vi "Destroy Request Events.vi"(8 "error in (no error)":errorcluster) -> (0 "error out":errorcluster)   [LabVIEW 2015, in "Tool Module.lvlib"]
doc: "Destroy the requests user events, even if there is an incoming error.\n\n<b>NOTE</b>: The contents of this VI are automatically generated and modified by the <b>Tools > Delacor > DQMH</b> utilities. Consider using those utilities instead of making your own modifications to this VI.\n_____\nBased on Delacor QMH Project Template 2.1.0.2."
uses:
  Tool Module.lvlib
panel:
  # "NOTE: The contents of this VI are automatically generated and modified by the Tools > Delacor > DQMH utilities. Consider using those utilities instead of making your own modifications to this VI."
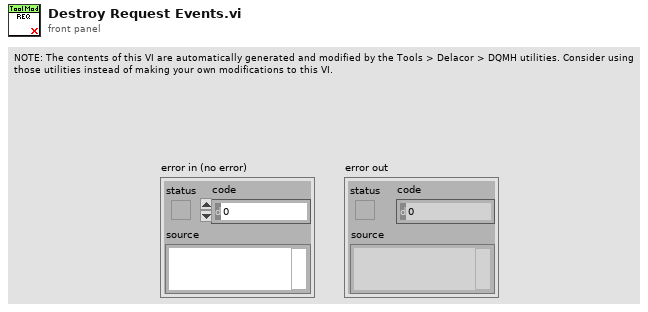
[diagram p1: front panel]
types:
  T1 = typedef "Tool Module.lvlib/Request Events--cluster.ctl" = cluster{"Stop Module":refnum<user-event>, "Show Panel":refnum<user-event>, "Hide Panel":refnum<user-event>, "Get Module Execution Status":refnum<user-event>, "Show Diagram":refnum<user-event>, "Test Trig 2":refnum<user-event>, "GOTO":refnum<user-event>, "Start Inspect":refnum<user-event>, "CONNECT":refnum<user-event>, "Get All Inspect Data":refnum<user-event>, "Get Inspection Limits":refnum<user-event>, "Set Inspection Limits":refnum<user-event>, "Update Status":refnum<user-event>, "Start Data Monitor":refnum<user-event>, "Get FPGA Setup Params":refnum<user-event>, "Set FPGA Setup Params":refnum<user-event>, "Set Tool Config":refnum<user-event>, "Get Tool Config":refnum<user-event>, "Set Integration Count":refnum<user-event>, "Set Laser Params":refnum<user-event>, "Get Mtrl Ctrl Reg":refnum<user-event>, "Commit Ctrl Reg":refnum<user-event>, "Set Event Logger":refnum<user-event>, "Write to File":refnum<user-event>, "Read from File":refnum<user-event>, "Set Device Temp Thresholds":refnum<user-event>, "Get Cycle Count":refnum<user-event>}
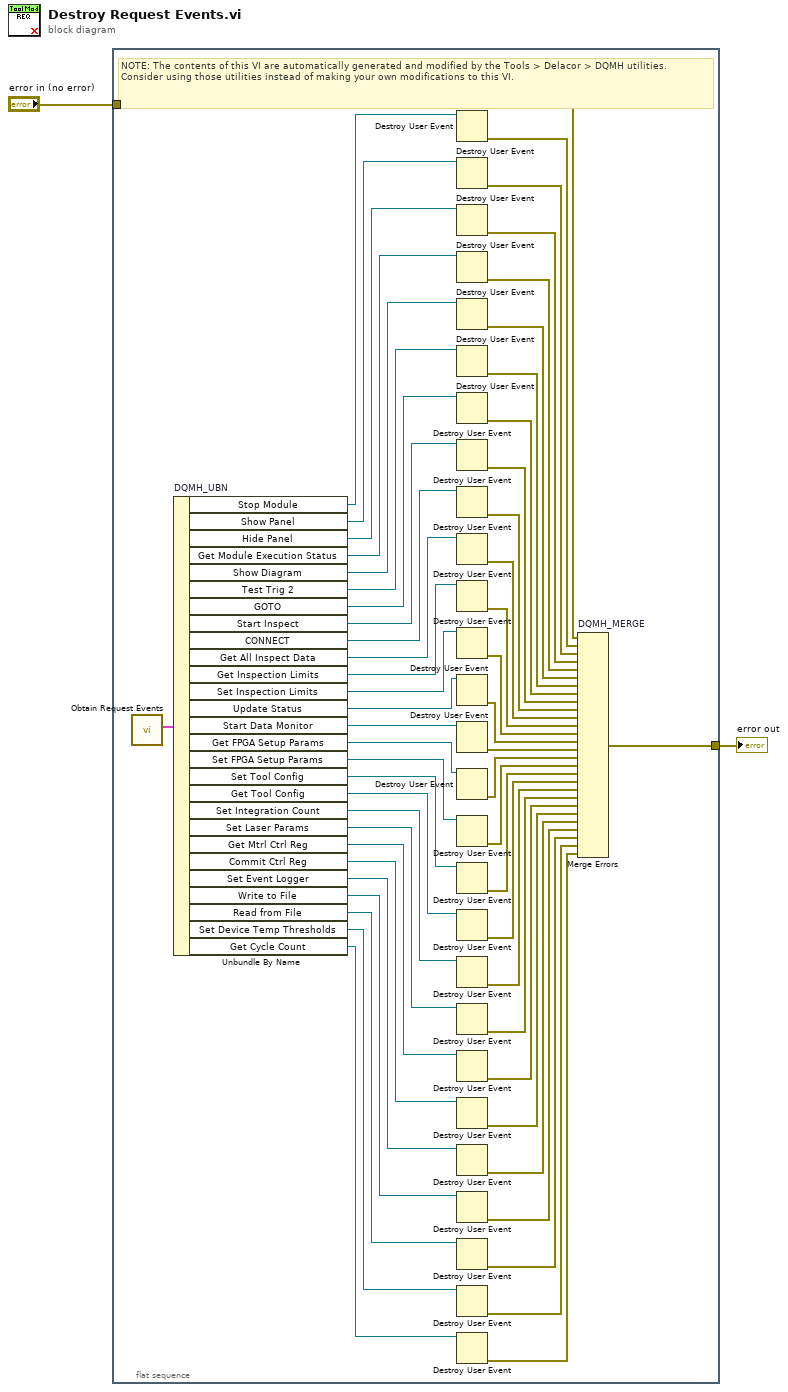
[diagram p0: block diagram]
diagram:
  n1 = flat-sequence {
    tunnel: [w58] -> w2
    tunnel: "error in (no error)" -> [w51]
    frame #0 {
      # "NOTE: The contents of this VI are automatically generated and modified by the Tools > Delacor > DQMH utilities. Consider using those utilities instead of making your own modifications to this VI."
      n2 = call "Obtain Request Events.vi"() -> ("Tool Module Request Events"=w57:T1)  [unwired: 10 in, 1 out]
      n3 = Unbundle By Name "DQMH_UBN"(w57) -> ("Stop Module"=w56:refnum<user-event>, "Show Panel"=w53:refnum<user-event>, "Hide Panel"=w52:refnum<user-event>, "Get Module Execution Status"=w49:refnum<user-event>, "Show Diagram"=w47:refnum<user-event>, "Test Trig 2"=w45:refnum<user-event>, "GOTO"=w43:refnum<user-event>, "Start Inspect"=w41:refnum<user-event>, "CONNECT"=w39:refnum<user-event>, "Get All Inspect Data"=w37:refnum<user-event>, "Get Inspection Limits"=w35:refnum<user-event>, "Set Inspection Limits"=w33:refnum<user-event>, "Update Status"=w31:refnum<user-event>, "Start Data Monitor"=w29:refnum<user-event>, "Get FPGA Setup Params"=w27:refnum<user-event>, "Set FPGA Setup Params"=w25:refnum<user-event>, "Set Tool Config"=w23:refnum<user-event>, "Get Tool Config"=w21:refnum<user-event>, "Set Integration Count"=w19:refnum<user-event>, "Set Laser Params"=w17:refnum<user-event>, "Get Mtrl Ctrl Reg"=w15:refnum<user-event>, "Commit Ctrl Reg"=w13:refnum<user-event>, "Set Event Logger"=w11:refnum<user-event>, "Write to File"=w9:refnum<user-event>, "Read from File"=w7:refnum<user-event>, "Set Device Temp Thresholds"=w5:refnum<user-event>, "Get Cycle Count"=w3:refnum<user-event>)
      n4 = Destroy User Event(user event=w56) -> (error out=w59:errorcluster)  [unwired: 1 in]
      n5 = Destroy User Event(user event=w53) -> (error out=w55:errorcluster)  [unwired: 1 in]
      n6 = Destroy User Event(user event=w52) -> (error out=w54:errorcluster)  [unwired: 1 in]
      n7 = Destroy User Event(user event=w49) -> (error out=w50:errorcluster)  [unwired: 1 in]
      n8 = Destroy User Event(user event=w47) -> (error out=w48:errorcluster)  [unwired: 1 in]
      n9 = Destroy User Event(user event=w45) -> (error out=w46:errorcluster)  [unwired: 1 in]
      n10 = Destroy User Event(user event=w43) -> (error out=w44:errorcluster)  [unwired: 1 in]
      n11 = Destroy User Event(user event=w41) -> (error out=w42:errorcluster)  [unwired: 1 in]
      n12 = Destroy User Event(user event=w39) -> (error out=w40:errorcluster)  [unwired: 1 in]
      n13 = Destroy User Event(user event=w37) -> (error out=w38:errorcluster)  [unwired: 1 in]
      n14 = Destroy User Event(user event=w35) -> (error out=w36:errorcluster)  [unwired: 1 in]
      n15 = Destroy User Event(user event=w33) -> (error out=w34:errorcluster)  [unwired: 1 in]
      n16 = Destroy User Event(user event=w31) -> (error out=w32:errorcluster)  [unwired: 1 in]
      n17 = Destroy User Event(user event=w29) -> (error out=w30:errorcluster)  [unwired: 1 in]
      n18 = Destroy User Event(user event=w27) -> (error out=w28:errorcluster)  [unwired: 1 in]
      n19 = Destroy User Event(user event=w25) -> (error out=w26:errorcluster)  [unwired: 1 in]
      n20 = Destroy User Event(user event=w23) -> (error out=w24:errorcluster)  [unwired: 1 in]
      n21 = Destroy User Event(user event=w21) -> (error out=w22:errorcluster)  [unwired: 1 in]
      n22 = Destroy User Event(user event=w19) -> (error out=w20:errorcluster)  [unwired: 1 in]
      n23 = Destroy User Event(user event=w17) -> (error out=w18:errorcluster)  [unwired: 1 in]
      n24 = Destroy User Event(user event=w15) -> (error out=w16:errorcluster)  [unwired: 1 in]
      n25 = Destroy User Event(user event=w13) -> (error out=w14:errorcluster)  [unwired: 1 in]
      n26 = Destroy User Event(user event=w11) -> (error out=w12:errorcluster)  [unwired: 1 in]
      n27 = Destroy User Event(user event=w9) -> (error out=w10:errorcluster)  [unwired: 1 in]
      n28 = Destroy User Event(user event=w7) -> (error out=w8:errorcluster)  [unwired: 1 in]
      n29 = Destroy User Event(user event=w5) -> (error out=w6:errorcluster)  [unwired: 1 in]
      n30 = Destroy User Event(user event=w3) -> (error out=w4:errorcluster)  [unwired: 1 in]
      n31 = Merge Errors "DQMH_MERGE"(w51, w59, w55, w54, w50, w48, w46, w44, w42, w40, w38, w36, w34, w32, w30, w28, w26, w24, w22, w20, w18, w16, w14, w12, w10, w8, w6, w4) -> (w58:errorcluster)
    }
  }
  "error out" <- w2
